vi "Control con Histeresis.vi"() -> ()   [LabVIEW 2020]
panel:
  out "Boolean":bool
  in  "Min":i32
  in  "Referencia":i32
  in  "Max":i32
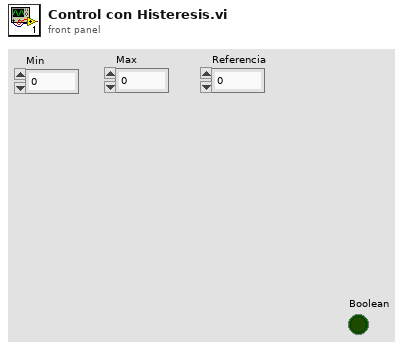
[diagram p1: front panel]
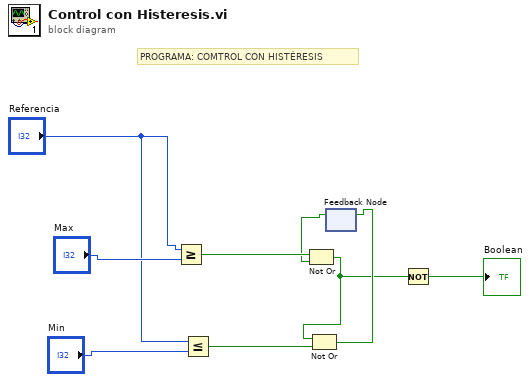
[diagram p0: block diagram]
diagram:
  # "PROGRAMA: COMTROL CON HISTÉRESIS"
  n1 = Greater Or Equal?(x="Referencia", y="Max") -> (x >= y?=w5:bool)
  n2 = Less Or Equal?(x="Referencia", y="Min") -> (x <= y?=w6:bool)
  n3 = feedback #1() -> (w4:bool)  [unwired: 1 in]
  n4 = Not Or(1:w4, 2:w5) -> (0:w2:bool)
  n5 = Not Or(1:w6, 2:w2) -> (0:w3:bool)
  n6 = feedback-in #1(w3) -> ()
  n7 = Not(x=w2) -> (.not. x?=→"Boolean":bool)
